vi "Set Group.vi"(10 "Group":string, 11 "Bark in":refnum<class "Bark.lvclass">) -> (3 "Bark out":refnum<class "Bark.lvclass">)   [LabVIEW 2016, in "Bark.lvlib" / "Bark.lvclass"]
uses:
  Bark.lvclass
  Bark.lvclass/Bark.ctl
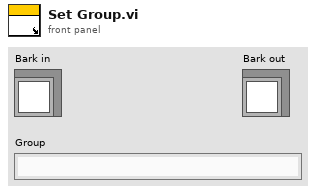
[diagram p1: front panel]
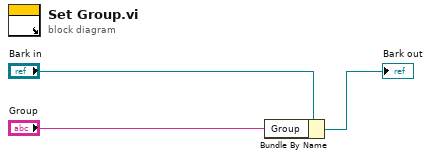
[diagram p0: block diagram]
diagram:
  n1 = Bundle By Name(cluster="Bark in", "Group"="Group") -> (→"Bark out":refnum<class "Bark.lvclass">)
